vi "FiltrosFIR.vi"() -> ()   [LabVIEW 2021]
uses:
  <vilib>/sound2/lvsound2.llb/Sound Data Format.ctl
  <vilib>/sound2/lvsound2.llb/Sampling Mode.ctl
  <vilib>/sound2/lvsound2.llb/Sound Output Set Volume (Single).vi
  <vilib>/sound2/lvsound2.llb/Sound Output Write (DBL).vi
  <vilib>/express/express analysis/Spectral/Block/exnSpectralBlock spectral measurements power poly.vi
  <vilib>/express/express analysis/Spectral/Block/exnSpectralBlock spectral measurements power array WFM.vi
  <vilib>/express/express analysis/Spectral/Block/exnSpectralBlock spectral measurements power DDT.vi
  <vilib>/express/express analysis/Spectral/XNode/ExpressSpectralMeasurementsBlockNode.xnode
panel:
  in  "Fecuencia de corte":dbl=100.0 caption="Lower Cut-Off"
  in  "Volumen":dbl(slide)=100.0 scale=0.0..100.0
  in  "Frecuencia 2":dbl(knob) scale=0.0..10000.0
  in  "Amplitud 2":dbl(knob) scale=0.0..100.0
  out "Sonido generado":waveform(dbl)[](graph)
  out "Señal filtrada":dynamicdata(graph)
  out "Espectro de las señales":cluster{"f0":dbl, "df":dbl, "magnitude":dbl[]}[](graph)
  in  "stop":bool
  in  "Amplitud 1":dbl(knob) scale=0.0..100.0
  in  "Frecuencia 1":dbl(knob) scale=0.0..5000.0
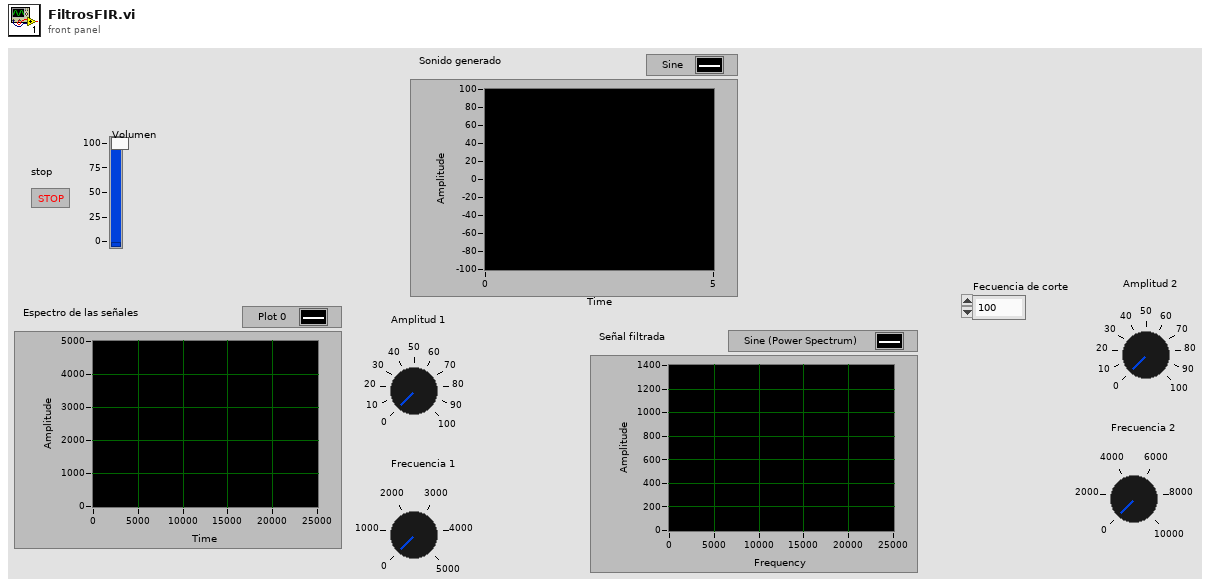
[diagram p1: front panel]
types:
  T1 = typedef "Sampling Mode.ctl" = i32
  T2 = typedef "Sound Data Format.ctl" = cluster{"sample rate (S/s)":dbl, "number of channels":i32, "bits per sample":i32}
  T3 = typedef "Sound Output Task ID.ctl" = u32
  T4 = cluster{"averaging mode":u16, "weighting mode":u16, "number of averages":u32}
  T5 = cluster{"dB On (F)":bool, "unwrap phase (F)":bool, "convert to degree (F)":bool}
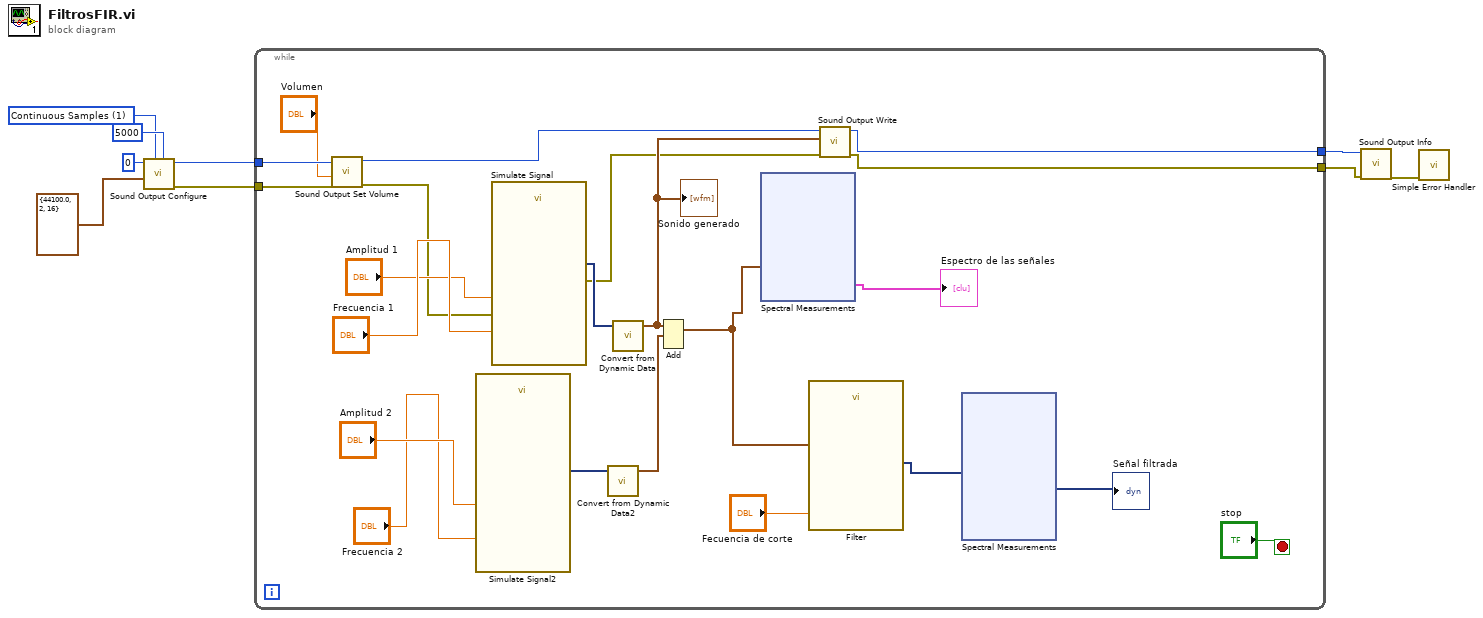
[diagram p0: block diagram]
diagram:
  w1 = T1 1 items=["Finite Samples", "Continuous Samples"] ("sample mode")
  n1 = call <vilib>:"Sound Output Configure.vi"("number of samples/ch"=5000, "sample mode"=w1, "sound format"=T2 {"sample rate (S/s)"=44100.0, "number of channels"=2, "bits per sample"=16}, "device ID"=u32 0) -> ("error out"=w5:errorcluster, "task ID"=w6:T3)  [unwired: 6 in]
  n2 = while {
    tunnel: [w18] -> w9
    tunnel: [w17] -> w7
    tunnel: w6 -> [w14]
    tunnel: w5 -> [w13]
    stop <- "stop" stop-if-true
    n3 = call-poly <vilib>:"Sound Output Set Volume.vi"("error in (no error)"=w13, "volume"="Volumen", "task ID"=w14) -> ("error out"=w16:errorcluster, "task ID out"=w19:T3)  [unwired: 7 in]
    n4 = call "Simulate Signal2"("Frequency"="Frecuencia 2", "Amplitude"="Amplitud 2") -> ("Triangle"=w25:dynamicdata)  [unwired: 12 in, 1 out]
    n5 = call "Simulate Signal"("Frequency"="Frecuencia 1", "Amplitude"="Amplitud 1", "error in (no error)"=w16) -> ("Sine"=w26:dynamicdata, "error out"=w15:errorcluster)  [unwired: 11 in]
    n6 = call "Convert from Dynamic Data2"("Dynamic Data Type"=w25) -> ("Array of Waveform"=w24:waveform(dbl)[])  [unwired: 3 in]
    n7 = call "Convert from Dynamic Data"("Dynamic Data Type"=w26) -> ("Array of Waveform"=w20:waveform(dbl)[])  [unwired: 3 in]
    "Sonido generado" <- w20
    n8 = Add(1:w24, 2:w20) -> (0:w12:waveform(dbl)[])  [unwired: 1 in, 1 out]
    n9 = xnode "Spectral Measurements"("Signals"=w12) -> ("Power Spectrum"=→"Espectro de las señales":cluster{"f0":dbl, "df":dbl, "magnitude":dbl[]}[])  [unwired: 1 in, 1 out]
    n10 = call "Filter"("Lower Cut-Off"="Fecuencia de corte", "Signal"=w12) -> ("Filtered Signal"=w23:dynamicdata)  [unwired: 8 in, 1 out]
    n11 = call-poly <vilib>:"Sound Output Write.vi"("error in (no error)"=w15, "data"=w20, "task ID"=w19) -> ("error out"=w17:errorcluster, "task ID out"=w18:T3)  [unwired: 7 in]
    n12 = xnode "Spectral Measurements"("Signals"=w23) -> ("Power Spectrum"=→"Señal filtrada":dynamicdata)  [unwired: 1 in, 1 out]
  }
  n13 = call <vilib>:"Sound Output Info.vi"("error in (no error)"=w7, "task ID"=w9) -> ("error out"=w8:errorcluster)  [unwired: 6 in, 3 out]
  n14 = call <vilib>:"Simple Error Handler.vi"("error in (no error)"=w8) -> ()  [unwired: 4 in, 5 out]
